vi "Main.vi"() -> ()   [LabVIEW 2017]
doc: "The myRIO Project template acquires acceleration data from the onboard accelerometer and displays the changes of acceleration values in a waveform chart."
uses:
  states.ctl
  Current Floor.ctl
  <vilib>/myRIO/Instrument Drivers/Onboard IO/DIO/typedefs/DIO Reference.ctl
  <vilib>/myRIO/Common/Instrument Driver Framework/Utilities/typedefs/myRIO Generic Hardware Reference.ctl
  <vilib>/myRIO/Common/Instrument Driver Framework/Utilities/typedefs/Hardware Version Enum.ctl
  <vilib>/myRIO/Common/Instrument Driver Framework/Utilities/typedefs/myRIO v1.0 Reference.ctl
  <vilib>/myRIO/Common/Instrument Driver Framework/Utilities/typedefs/Generic FPGA Reference.ctl
  <vilib>/myRIO/Common/Instrument Driver Framework/myRIO v1.0/DIO/typedefs/DIO Channels List.ctl
  <vilib>/myRIO/Common/Instrument Driver Framework/myRIO v1.0/DIO/typedefs/DIO Channels Enum.ctl
  <vilib>/userdefined/High Color/nirio_resource_hc.ctl
  <vilib>/myRIO/Common/Instrument Driver Framework/Utilities/vis/Is FPGA Ref Available.vi
  <vilib>/myRIO/Common/Instrument Driver Framework/myRIO v1.0/DIO/vis/myRIO v1.1 Open DIO.vi
  <vilib>/myRIO/Instrument Drivers/Onboard IO/DIO/vis/Read.vi
  <vilib>/myRIO/Instrument Drivers/Onboard IO/DIO/vis/Write.vi
  <vilib>/myRIO/Common/Instrument Driver Framework/Utilities/vis/Validate Channels.vi
  <vilib>/myRIO/Common/Instrument Driver Framework/myRIO v1.0/DIO/vis/myRIO v1.0 Reserve DIO.vi
  <vilib>/myRIO/Common/Instrument Driver Framework/myRIO v1.0/Resource Manager/vis/myRIO v1.0 Reserve Channel List.vi
  <vilib>/myRIO/Common/Instrument Driver Framework/myRIO v1.0/DIO/vis/myRIO v1.0 Build MUX Configuration DIO.vi
  <vilib>/myRIO/Common/Instrument Driver Framework/myRIO v1.0/Resource Manager/vis/myRIO v1.0 Reserve Channel.vi
  <vilib>/myRIO/Common/Instrument Driver Framework/myRIO v1.0/Resource Manager/vis/myRIO v1.0 Unreserve Channel.vi
  <vilib>/myRIO/Common/Instrument Driver Framework/myRIO v1.0/Resource Manager/vis/myRIO v1.0 Create Configuration List.vi
  <vilib>/myRIO/Common/Instrument Driver Framework/myRIO v1.0/Resource Manager/vis/myRIO v1.0 Build Mutex Name.vi
  <vilib>/Utility/VariantDataType/GetNumericInfo.vi
  <vilib>/Utility/error.llb/Error Cluster From Error Code.vi
  <vilib>/myRIO/Common/Instrument Driver Framework/myRIO v1.0/myRIO v1.1 Open.vi
  <vilib>/myRIO/Common/Instrument Driver Framework/Utilities/vis/IO Manager.vi
  <vilib>/myRIO/Common/Instrument Driver Framework/Utilities/vis/Configuration Manager.vi
  <vilib>/myRIO/Common/Instrument Driver Framework/myRIO v1.0/Resource Manager/vis/myRIO v1.0 Configure IO.vi
  <vilib>/myRIO/Common/Instrument Driver Framework/myRIO v1.0/myRIO v1.0 Close.vi
  <vilib>/myRIO/Common/Instrument Driver Framework/myRIO v1.0/DIO/vis/myRIO v1.0 Read DIO.vi
  <vilib>/myRIO/Common/Instrument Driver Framework/myRIO v1.0/DIO/vis/myRIO v1.0 Write DIO.vi
  <vilib>/myRIO/Express VI/Onboard IO/DI/DI Express VI.xnode
  <vilib>/myRIO/Instrument Drivers/Onboard IO/DIO/vis/myRIO DIO Open.xnode
  <vilib>/myRIO/Express VI/Onboard Devices/LED/LED Express VI.xnode
  <vilib>/myRIO/Instrument Drivers/Onboard IO/DIO/DIO.lvlib
panel:
  out "At Ground From Drop":i32
  out "At Floor 2":i32
  out "At Floor 1":i32
  out "At Ground":i32
  in  "Stop Button":bool
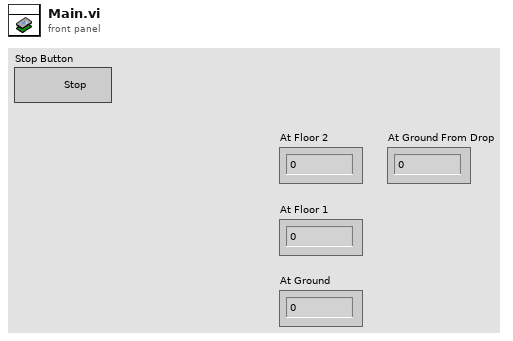
[diagram p1: front panel]
types:
  T1 = typedef "Current Floor.ctl" = enum16{"Ground Floor", "Floor 1", "Floor 2"}
  T2 = typedef "states.ctl" = enum16{"waiting for command", "go to ground floor", "go to floor 1", "go to floor 2", "drop cart"}
  T3 = typedef "DIO.lvlib/DIO Reference.ctl" = cluster{"myRIO Reference":T4, "DIO Channels List":T8}
  T4 = typedef "myRIO Generic Hardware Reference.ctl" = cluster{"myRIO Model":T5, "myRIO Hardware Reference":T6}
  T5 = typedef "Hardware Version Enum.ctl" = enum16{"Unknown", "myRIO-1900", "myRIO-1950", "roboRIO", "NI ELVIS RIO CM"}
  T6 = typedef "myRIO v1.0 Reference.ctl" = cluster{"Generic FPGA Reference":T7, "Allow multiple opens":bool}
  T7 = typedef "Generic FPGA Reference.ctl" = refnum<k20>
  T8 = typedef "DIO Channels List.ctl" = T9[]
  T9 = typedef "DIO Channels Enum.ctl" = enum16{"Not Connected", "C/DIO0", "C/DIO1", "C/DIO2", "C/DIO3", "C/DIO4", "C/DIO5", "C/DIO6", "C/DIO7", "A/DIO0", "A/DIO1", "A/DIO2", "A/DIO3", "A/DIO4", "A/DIO5", "A/DIO6", "A/DIO7", "A/DIO8", "A/DIO9", "A/DIO10", "A/DIO11", "A/DIO12", "A/DIO13", "A/DIO14", "A/DIO15", "B/DIO0", "B/DIO1", "B/DIO2", "B/DIO3", "B/DIO4", "B/DIO5", "B/DIO6", "B/DIO7", "B/DIO8", "B/DIO9", "B/DIO10", "B/DIO11", "B/DIO12", "B/DIO13", "B/DIO14", "B/DIO15", "LED0", "LED1", "LED2", "LED3", "Button0", "DIO/DIO0", "DIO/DIO1", "DIO/DIO2", "DIO/DIO3", "DIO/DIO4", "DIO/DIO5", "DIO/DIO6", "DIO/DIO7", "DIO/DIO8", "DIO/DIO9", "SPI/CS0", "SPI/CS1", "SPI/CS2", "SPI/CS3", "LED RADIO (Green)", "LED RADIO (Red)", "LED COMM (Green)", "LED COMM (Red)", "LED MODE (Green)", "LED MODE (Red)"}
  T10 = typedef "nirio_resource_hc.ctl" = tag
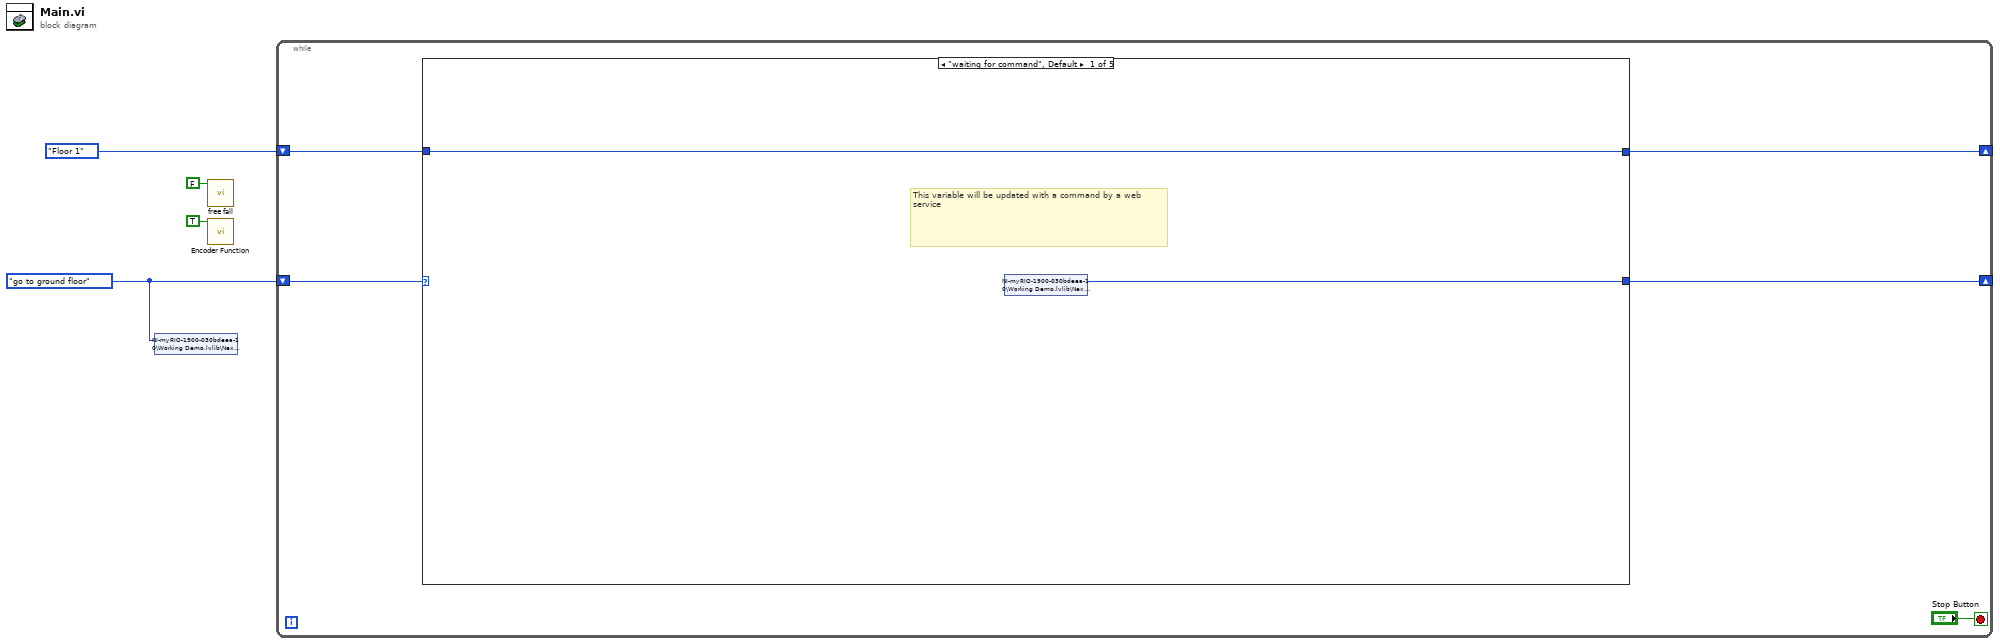
[diagram p0: block diagram]
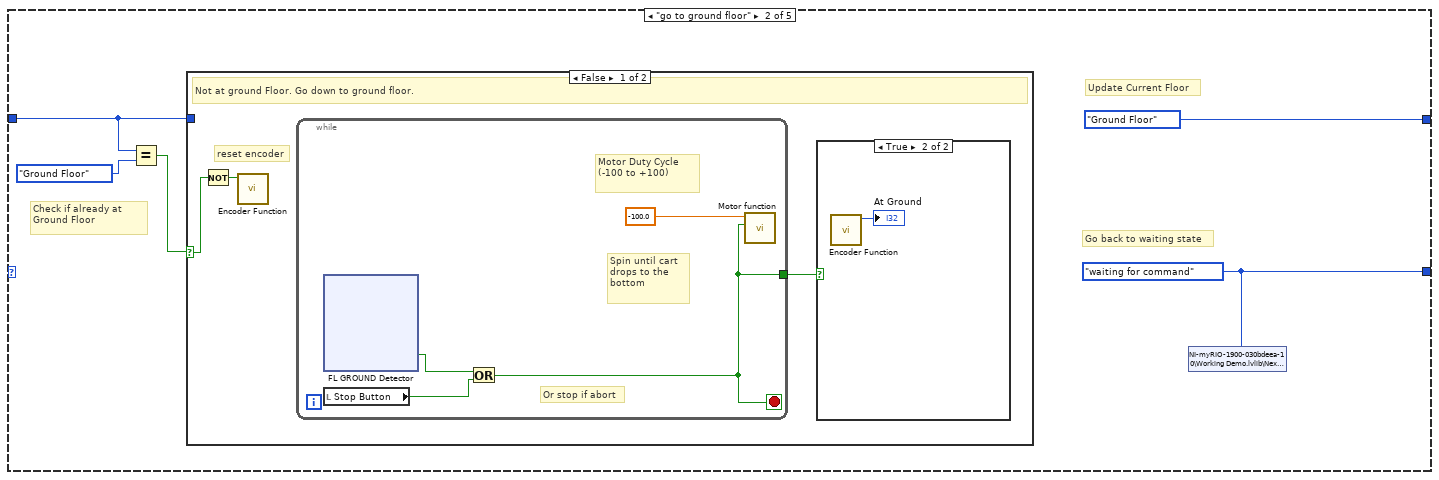
[diagram p2: hidden frame]
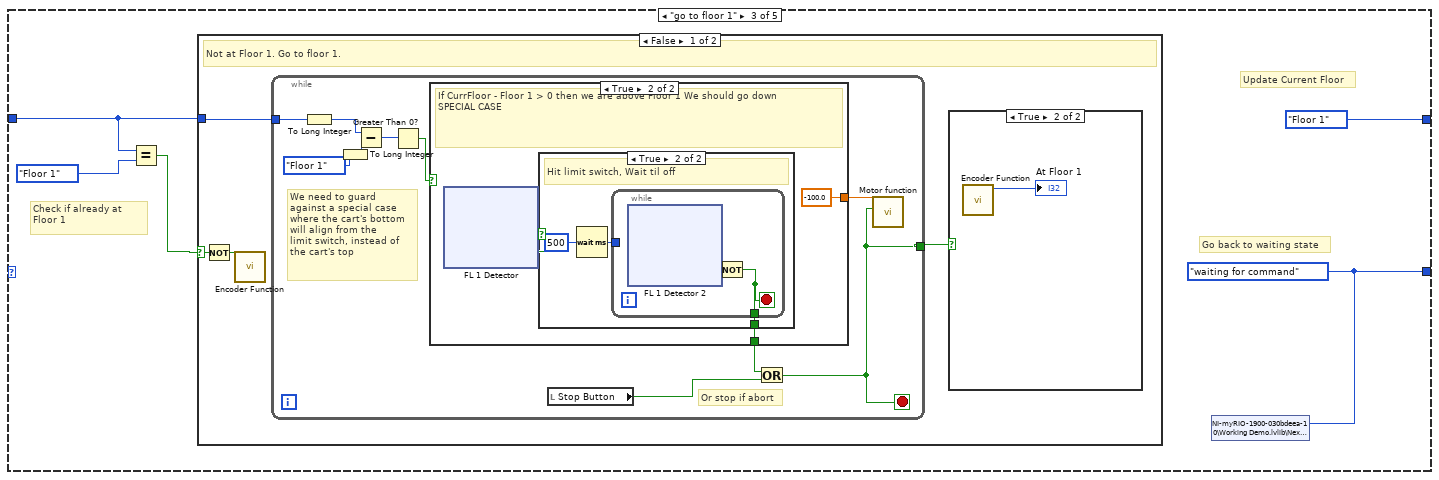
[diagram p5: hidden frame]
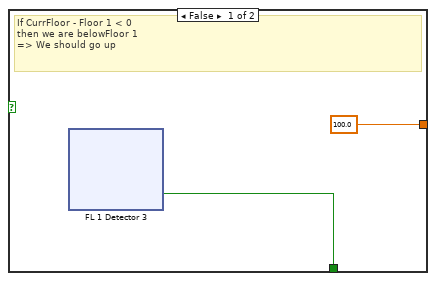
[diagram p7: hidden frame]
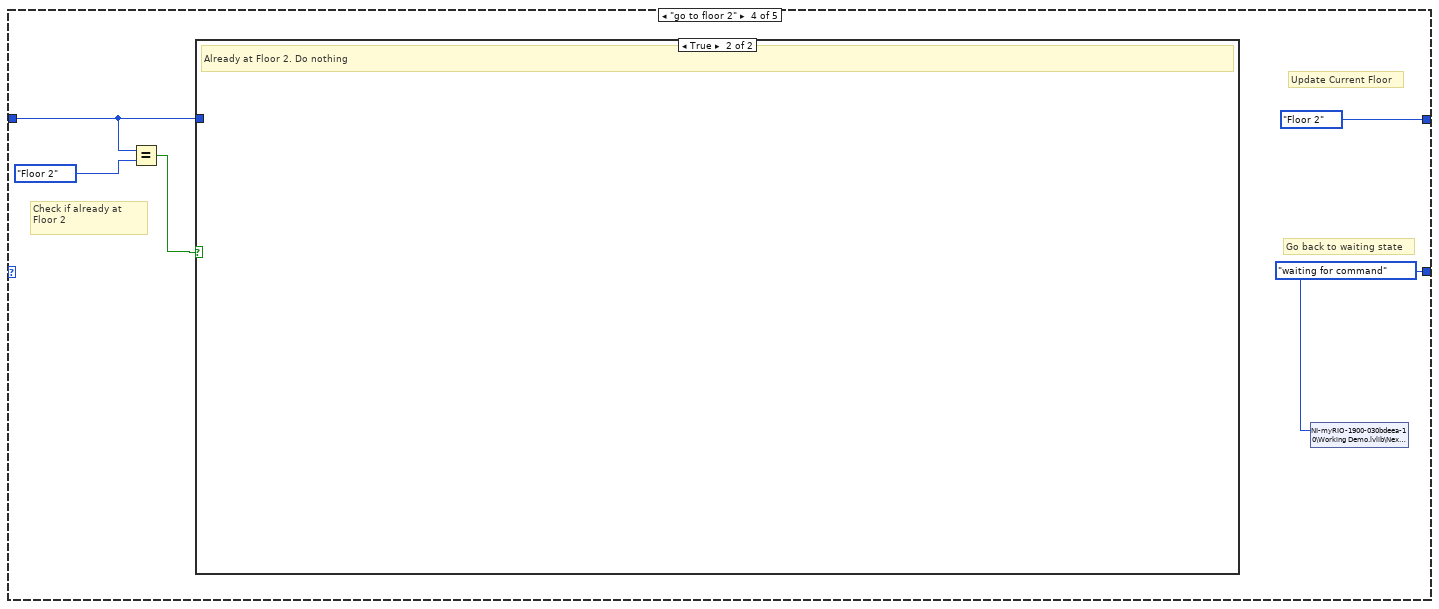
[diagram p10: hidden frame]
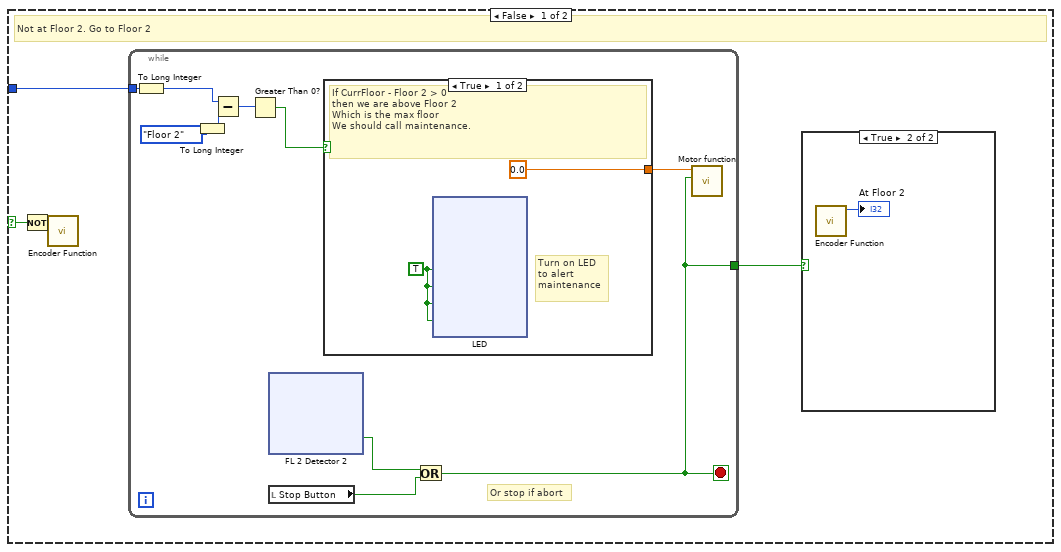
[diagram p11: hidden frame]
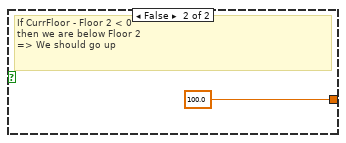
[diagram p13: hidden frame]
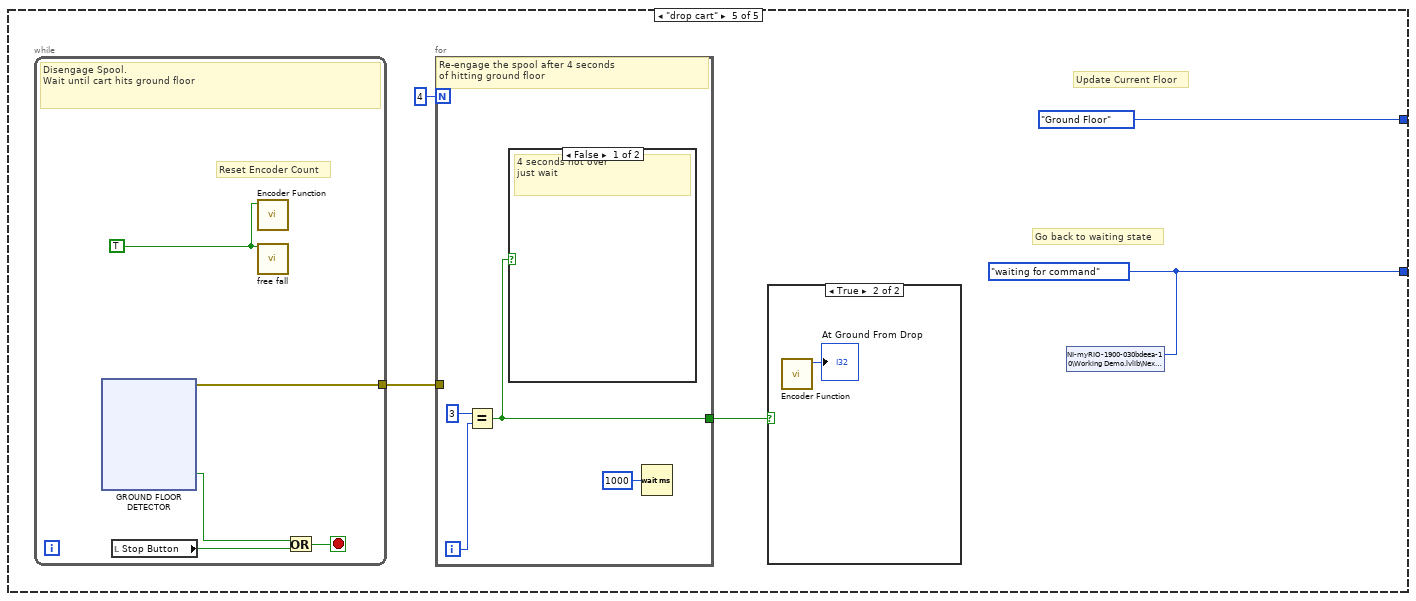
[diagram p14: hidden frame]
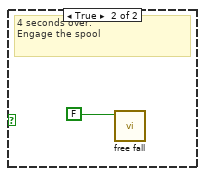
[diagram p16: hidden frame]
diagram:
  w3 = states."go to ground floor"
  n1 = shared-variable "NI-myRIO-1900-030bdeea-10\\Working Demo.lvlib\\Next State"(w3) -> ()  [unwired: 1 in, 1 out]
  n2 = call "free fall.vi"("Freefall Button"=FALSE) -> ()  [unwired: 11 in]
  n3 = call "Encoder Function.vi"("Reset Counter in"=TRUE) -> ()  [unwired: 9 in, 2 out]
  n4 = while {
    shift-right: [w7] -> _
    shift-left: w3 -> [w8]
    shift-right: [w5] -> _
    shift-left: Current_Floor."Floor 1" -> [w6]
    stop <- "Stop Button" stop-if-true
    n5 = case shown="\"waiting for command\", Default" w8 {
      tunnel: [w11 w12 w60 w195 w292] -> w7
      tunnel: w6 -> [w10 w13 w61 w196 _]
      tunnel: [w10 Current_Floor."Ground Floor" Current_Floor."Floor 1" Current_Floor."Floor 2" Current_Floor."Ground Floor"] -> w5
      frame "waiting for command", Default {
        # "This variable will be updated with a command by a web service"
        n6 = shared-variable "NI-myRIO-1900-030bdeea-10\\Working Demo.lvlib\\Next State"() -> (w11:T2)  [unwired: 1 in, 1 out]
      }
      frame "go to ground floor" {
        w12 = states."waiting for command"
        # "Update Current Floor"
        # "Go back to waiting state"
        # "Check if already at Ground Floor"
        n7 = Equal?(x=w13, y=Current_Floor."Ground Floor") -> (x = y?=w14:bool)
        n8 = case shown="False" w14 {
          selector: w14 -> [w19 _]
          tunnel: w13 -> [_ _]
          frame False {
            # "reset encoder"
            # "Not at ground Floor. Go down to ground floor."
            n9 = Not(x=w19) -> (.not. x?=w17:bool)
            n10 = call "Encoder Function.vi"("Reset Counter in"=w17) -> ()  [unwired: 9 in, 2 out]
            n11 = while {
              tunnel: [w21] -> w18
              stop <- w21 stop-if-true
              # "Motor Duty Cycle (-100 to +100)"
              # "Or stop if abort"
              # "Spin until cart drops to the bottom"
              n12 = xnode "FL GROUND Detector"() -> ("Ground Floor OPTLIMSW (B/DIO3 (Pin 17))"=w22:bool)  [unwired: 1 in, 1 out]
              n13 = local read "Stop Button"() -> (w24:bool)
              n14 = Or(x=w22, y=w24) -> (x .or. y?=w21:bool)
              n15 = call "Motor function.vi"("Stop VI"=w21, "Duty Cycle (-100 to +100)"=-100.0) -> ()  [unwired: 10 in]
            }
            n16 = case shown="True" w18 {
              frame False {
              }
              frame True {
                n17 = call "Encoder Function.vi"() -> ("Counter Value 2"=→"At Ground":i32)  [unwired: 10 in, 1 out]
              }
            }
          }
          frame True {
            # "Already at Ground Floor. Do nothing"
          }
        }
        n18 = shared-variable "NI-myRIO-1900-030bdeea-10\\Working Demo.lvlib\\Next State"(w12) -> ()  [unwired: 1 in, 1 out]
      }
      frame "go to floor 1" {
        w60 = states."waiting for command"
        # "Update Current Floor"
        # "Go back to waiting state"
        # "Check if already at Floor 1"
        n19 = Equal?(x=w61, y=Current_Floor."Floor 1") -> (x = y?=w62:bool)
        n20 = case shown="False" w62 {
          selector: w62 -> [w67 _]
          tunnel: w61 -> [w68 _]
          frame False {
            # "Not at Floor 1. Go to floor 1."
            n21 = Not(x=w67) -> (.not. x?=w66:bool)
            n22 = call "Encoder Function.vi"("Reset Counter in"=w66) -> ()  [unwired: 9 in, 2 out]
            n23 = while {
              tunnel: w68 -> [w78]
              tunnel: [w73] -> w65
              stop <- w73 stop-if-true
              # "We need to guard\nagainst a special case\nwhere the cart's bottom\nwill align from the\nlimit switch, instead of\nthe cart's top"
              # "Or stop if abort"
              n24 = To Long Integer(number=w78) -> (32bit integer=w75:i32)
              n25 = To Long Integer(number=Current_Floor."Floor 1") -> (32bit integer=w74:i32)
              n26 = Subtract(x=w75, y=w74) -> (x-y=w76:i32)
              n27 = Greater Than 0?(x=w76) -> (x > 0?=w72:bool)
              n28 = case shown="True" w72 {
                tunnel: [w81 w118] -> w71
                tunnel: [100.0 -100.0] -> w70
                frame False {
                  # "If CurrFloor - Floor 1 < 0\nthen we are belowFloor 1\n=> We should go up"
                  n29 = xnode "FL 1 Detector 3"() -> ("Floor 1 OPTLIMSW (B/DIO1 (Pin 13))"=w81:bool)  [unwired: 1 in, 1 out]
                }
                frame True {
                  # "If CurrFloor - Floor 1 > 0 then we are above Floor 1 We should go down\nSPECIAL CASE"
                  n30 = xnode "FL 1 Detector"() -> ("Floor 1 OPTLIMSW (B/DIO1 (Pin 13))"=w119:bool)  [unwired: 1 in, 1 out]
                  n31 = case shown="True" w119 {
                    tunnel: [_ w120] -> w118
                    frame False {
                    }
                    frame True {
                      # "Hit limit switch, Wait til off"
                      n32 = Wait (ms)(milliseconds to wait=u32 500) -> (millisecond timer value=w121:u32)
                      n33 = while {
                        tunnel: w121 -> [_]
                        tunnel: [w123] -> w120
                        stop <- w123 stop-if-true
                        n34 = xnode "FL 1 Detector 2"() -> ("Floor 1 OPTLIMSW (B/DIO1 (Pin 13))"=w124:bool)  [unwired: 1 in, 1 out]
                        n35 = Not(x=w124) -> (.not. x?=w123:bool)
                      }
                    }
                  }
                }
              }
              n36 = local read "Stop Button"() -> (w79:bool)
              n37 = Or(x=w71, y=w79) -> (x .or. y?=w73:bool)
              n38 = call "Motor function.vi"("Stop VI"=w73, "Duty Cycle (-100 to +100)"=w70) -> ()  [unwired: 10 in]
            }
            n39 = case shown="True" w65 {
              frame False {
              }
              frame True {
                n40 = call "Encoder Function.vi"() -> ("Counter Value 2"=→"At Floor 1":i32)  [unwired: 10 in, 1 out]
              }
            }
          }
          frame True {
            # "Already at Floor 1. Do nothing"
          }
        }
        n41 = shared-variable "NI-myRIO-1900-030bdeea-10\\Working Demo.lvlib\\Next State"(w60) -> ()  [unwired: 1 in, 1 out]
      }
      frame "go to floor 2" {
        w195 = states."waiting for command"
        # "Update Current Floor"
        # "Go back to waiting state"
        # "Check if already at Floor 2"
        n42 = Equal?(x=w196, y=Current_Floor."Floor 2") -> (x = y?=w197:bool)
        n43 = case shown="True" w197 {
          selector: w197 -> [w201 _]
          tunnel: w196 -> [w203 _]
          frame False {
            # "Not at Floor 2. Go to Floor 2"
            n44 = Not(x=w201) -> (.not. x?=w200:bool)
            n45 = call "Encoder Function.vi"("Reset Counter in"=w200) -> ()  [unwired: 9 in, 2 out]
            n46 = while {
              tunnel: w203 -> [w213]
              tunnel: [w205] -> w202
              stop <- w205 stop-if-true
              # "Or stop if abort"
              n47 = To Long Integer(number=w213) -> (32bit integer=w208:i32)
              n48 = To Long Integer(number=Current_Floor."Floor 2") -> (32bit integer=w207:i32)
              n49 = Subtract(x=w208, y=w207) -> (x-y=w211:i32)
              n50 = Greater Than 0?(x=w211) -> (x > 0?=w210:bool)
              n51 = xnode "FL 2 Detector 2"() -> ("Floor 2 OPTLIMSW (B/DIO2 (Pin 15))"=w206:bool)  [unwired: 1 in, 1 out]
              n52 = local read "Stop Button"() -> (w214:bool)
              n53 = case shown="True" w210 {
                tunnel: [0.0 ("Duty Cycle (-100 to +100)") 100.0 ("Duty Cycle (-100 to +100)")] -> w209
                frame True {
                  w215 = TRUE ("LED0")
                  # "Turn on LED\nto alert\nmaintenance"
                  # "If CurrFloor - Floor 2 > 0\nthen we are above Floor 2\nWhich is the max floor\nWe should call maintenance."
                  n54 = xnode "LED"("LED0"=w215, "LED1"=w215, "LED2"=w215, "LED3"=w215) -> ()  [unwired: 1 in, 1 out]
                }
                frame False {
                  # "If CurrFloor - Floor 2 < 0\nthen we are below Floor 2\n=> We should go up"
                }
              }
              n55 = Or(x=w206, y=w214) -> (x .or. y?=w205:bool)
              n56 = call "Motor function.vi"("Stop VI"=w205, "Duty Cycle (-100 to +100)"=w209) -> ()  [unwired: 10 in]
            }
            n57 = case shown="True" w202 {
              frame False {
              }
              frame True {
                n58 = call "Encoder Function.vi"() -> ("Counter Value 2"=→"At Floor 2":i32)  [unwired: 10 in, 1 out]
              }
            }
          }
          frame True {
            # "Already at Floor 2. Do nothing"
          }
        }
        n59 = shared-variable "NI-myRIO-1900-030bdeea-10\\Working Demo.lvlib\\Next State"(w195) -> ()  [unwired: 1 in, 1 out]
      }
      frame "drop cart" {
        w292 = states."waiting for command"
        # "Update Current Floor"
        # "Go back to waiting state"
        n60 = while {
          tunnel: [w304] -> w294
          stop <- w305 stop-if-true
          w302 = TRUE
          # "Reset Encoder Count"
          # "Disengage Spool.\nWait until cart hits ground floor"
          n61 = xnode "GROUND FLOOR DETECTOR"() -> ("GROUND FL OPTLIMSW (B/DIO3 (Pin 17))"=w303:bool, "error out"=w304:errorcluster)  [unwired: 1 in]
          n62 = local read "Stop Button"() -> (w306:bool)
          n63 = call "Encoder Function.vi"("Reset Counter in"=w302) -> ()  [unwired: 9 in, 2 out]
          n64 = call "free fall.vi"("Freefall Button"=w302) -> ()  [unwired: 11 in]
          n65 = Or(x=w303, y=w306) -> (x .or. y?=w305:bool)
        }
        n66 = for {
          N: 4 -> [_]
          tunnel: w294 -> [_]
          tunnel: [w297] -> w291
          i -> [w300]
          # "Re-engage the spool after 4 seconds \nof hitting ground floor"
          n67 = Equal?(x=3, y=w300) -> (x = y?=w297:bool)
          n68 = case shown="False" w297 {
            frame False {
              # "4 seconds not over\njust wait"
            }
            frame True {
              # "4 seconds over.\nEngage the spool"
              n69 = call "free fall.vi"("Freefall Button"=FALSE) -> ()  [unwired: 11 in]
            }
          }
          n70 = Wait (ms)(milliseconds to wait=u32 1000) -> ()  [unwired: 1 out]
        }
        n71 = case shown="True" w291 {
          frame False {
          }
          frame True {
            n72 = call "Encoder Function.vi"() -> ("Counter Value 2"=→"At Ground From Drop":i32)  [unwired: 10 in, 1 out]
          }
        }
        n73 = shared-variable "NI-myRIO-1900-030bdeea-10\\Working Demo.lvlib\\Next State"(w292) -> ()  [unwired: 1 in, 1 out]
      }
    }
  }
